vi "Actor Core.vi"(8 "error in":errorcluster caption="错误输入", 11 "Custor in":refnum<class "Custor.lvclass"> caption="操作者输入") -> (0 "error out":errorcluster caption="错误输出", 3 "Actor out":refnum<class "Actor.lvclass"> caption="操作者输出")   [LabVIEW 2024, in "Custor.lvlib" / "Custor.lvclass"]
doc: "<p>（<strong>文件名</strong>：<span class=\"dnl\">Actor Framework.lvlib:Actor.lvclass:Actor Core.vi</span>)</p>\n<p>接收发送至操作者的消息，响应消息并处理可能导致操作者关闭的错误。</p>\n<p>子孙类重写该VI，使操作者完成特定的任务。使用<a href=\"nihelplauncher://docs/csh?context=lvcore_glang_udclass\">调用父类方法</a>节点实现重写。</p>"
uses:
  Custor.lvclass
  <vilib>/ActorFramework/Actor/Actor.lvclass
  Custor.lvclass/Custor.ctl
  <vilib>/ActorFramework/Actor/Actor.lvclass/Actor.ctl
  <vilib>/ActorFramework/Message Enqueuer/Message Enqueuer.lvclass/Message Enqueuer.ctl
  <vilib>/ActorFramework/Message Enqueuer/Init from Existing Queue.vi
  <vilib>/ActorFramework/Message Enqueuer/Enqueue.vi
  <vilib>/ActorFramework/Stop Msg/Stop Msg.lvclass
  <vilib>/ActorFramework/Message Priority Queue/Priority Enqueue.vi
  <vilib>/ActorFramework/Message Enqueuer/Message Enqueuer.lvclass
  C:/Program Files (x86)/National Instruments/LabVIEW 2024/vi.lib/ActorFramework/Actor/Actor.lvclass
panel:
  out "Log":string
  out "Receive":string
  in  "Send":bool
  in  "Msg":string
  # "Custor"
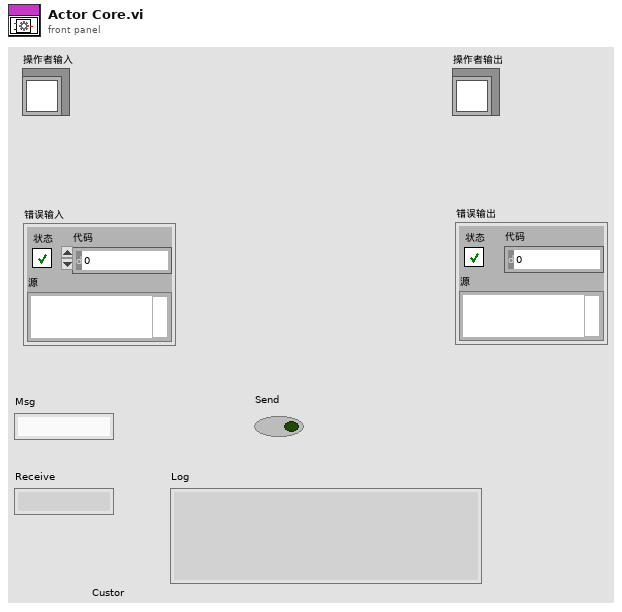
[diagram p1: front panel]
types:
  T1 = enum32{"Invalid", "Standard", "Closed", "Hidden", "Minimized", "Maximized"}
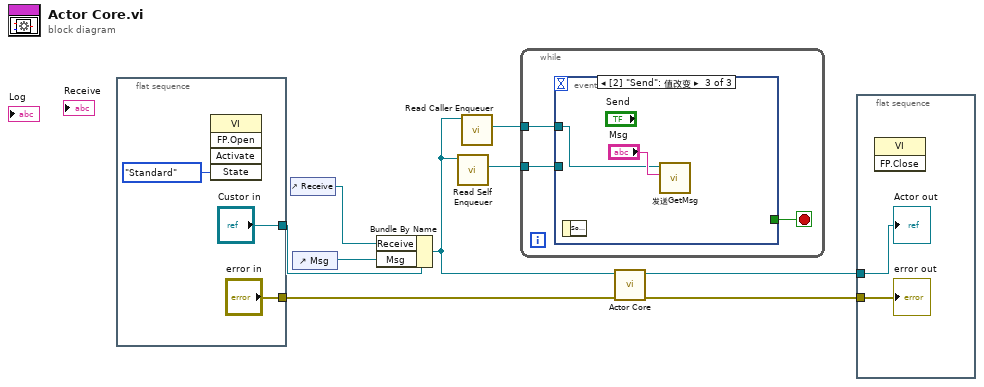
[diagram p0: block diagram]
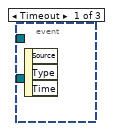
[diagram p2: hidden frame]
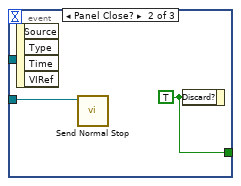
[diagram p3: hidden frame]
diagram:
  n1 = flat-sequence {
    tunnel: ["error in"] -> w7
    tunnel: ["Custor in"] -> w6
    frame #0 {
      n2 = invoke class="VI" method="FP.Open"("State"=T1."Standard" ("状态")) -> ()  [unwired: 4 in, 5 out]
    }
  }
  n3 = control-ref of="Receive"() -> (w4:refnum<vi>)
  n4 = control-ref of="Msg"() -> (w5:refnum<vi>)
  n5 = Bundle By Name(cluster=w6, "Receive"=w4, "Msg"=w5) -> (w2:refnum<class "Custor.lvclass">)
  n6 = call <vilib>:"Read Self Enqueuer.vi"("Actor"=w2) -> ("Self Enqueuer"=w3:refnum<class "Message Enqueuer.lvclass">)  [unwired: 10 in]
  n7 = call <vilib>:"Read Caller Enqueuer.vi"("Actor"=w2) -> ("Caller Enqueuer"=w1:refnum<class "Message Enqueuer.lvclass">)  [unwired: 10 in]
  n8 = while {
    tunnel: w3 -> [w15]
    tunnel: w1 -> [w13]
    stop <- w14 stop-if-true
    n9 = event shown="[2] \"Send\": 值改变" {
      selector: _ -> [_ _ _]
      dyn-events: _ -> [_ _ _]
      timeout: _ -> [_ _ _]
      tunnel: w15 -> [_ w17 _]
      tunnel: [_ w16 _] -> w14
      tunnel: w13 -> [_ _ w18]
      event Timeout {
        n10 = event-data() -> ()  [unwired: 1 in, 3 out]
      }
      event Panel Close? {
        w16 = TRUE ("放弃？")
        n11 = event-data() -> ()  [unwired: 1 in, 4 out]
        n12 = call <vilib>:"Send Normal Stop.vi"("Message Enqueuer"=w17) -> ()  [unwired: 10 in, 1 out]
        n13 = event-data("Discard?"=w16) -> ()  [unwired: 1 in, 1 out]
      }
      event "Send": Value Change {
        n14 = event-data() -> ()  [unwired: 1 in, 1 out]
        n15 = call "发送GetMsg.vi"("Receive"="Msg", "Message Enqueuer"=w18) -> ()  [unwired: 8 in, 2 out]
      }
    }
  }
  n16 = call-parent "Actor Core.vi"("error in"=w7, "Actor in"=w2) -> ("error out"=w9:errorcluster, "Actor out"=w8:refnum<class "Actor.lvclass">)  [unwired: 8 in]
  n17 = flat-sequence {
    tunnel: w9 -> [w21]
    tunnel: w8 -> [w20]
    frame #0 {
      n18 = invoke class="VI" method="FP.Close"() -> ()  [unwired: 3 in, 3 out]
      "error out" <- w21
      "Actor out" <- w20
    }
  }
